vi "FPGAinit.vi"(4 "Testpulse Cluster":T3={"Master Pulser On/Off"=FALSE, "Testpulse Turnaround Time (samples)"=14, "Pulse Separation (samples)"=0, "Pulse duration (samples)"=0}, 5 "DAQ Info Cluster":T2={"Data Chunks per File"=1000, "Samples per Waveform"=95, "Pretrigger Samples"=15, "circular buffer length (samples)"=1000, "Waveforms per Data Chunk"=5000} {"Waveforms per Data Chunk" format="%.2p"}, 6 "Channel Cluster":T1={"det_type"=["", "", "", "", "", "", "", ""], "Serial numbers"=["", "", "", "", "", "", "", ""], "Sources"=["", "", "", "", "", "", "", ""], "Trigger level"=[4000, 4000, 4000, 4000, 4000, 4000, 4000, 4000], "Data Record On/Off"=[FALSE, FALSE, FALSE, FALSE, FALSE, FALSE, FALSE, FALSE], "Number of Channels"=8}, 7 "General Cluster":cluster{"Location":i16} {"Location" items=["Purdue", "NIKHEF", "Zurich", "???"]}, 8 "error in":errorcluster, 11 "FPGA VI Reference In":refnum<k20>) -> (0 "error out":errorcluster, 3 "FPGA VI Reference Out":refnum<k20>)   [LabVIEW 2012]
uses:
  <vilib>/FPGAPlugInAG/Dynamic/niLvFpga_Reset_Dynamic.vi
  <vilib>/Utility/error.llb/Error Cluster From Error Code.vi
  <vilib>/LabVIEW Targets/FPGA/FlexRIO/CustomFPGAMethods/79XXR_Method_IOModuleStatusImpl.vi
  <vilib>/FPGAPlugInAG/Dynamic/niLvFpga_Run_Dynamic.vi
  <vilib>/rvi/errors/niLvFpgaAdjustHostInterfaceError.vi
  <vilib>/rvi/interface/nirviMethod/nirviMethod.xnode
  <vilib>/rvi/interface/nirviReadWriteControl/nirviReadWriteControl.xnode
  <vilib>/rvi/errors/niLvFpgaMergeErrorWithErrorCode.vi
  <vilib>/rvi/interface/Simulation/niFpgaSimulationCallBeginRW.vi
  NiFpgaLv.dll
  <vilib>/FPGAPlugInAG/Dynamic/niLvFpga_ConfigureFifo_Dynamic.vi
  <vilib>/FPGAPlugInAG/Dynamic/niLvFpga_StartFifo_Dynamic.vi
panel:
  # "Channel 0"
  # "Channel 1"
  # "Channel 2"
  # "Channel 3"
  # "Channel 4"
  # "Channel 5"
  # "Channel 6"
  # "Channel 7"
  # "Waveform/Data Chunk information"
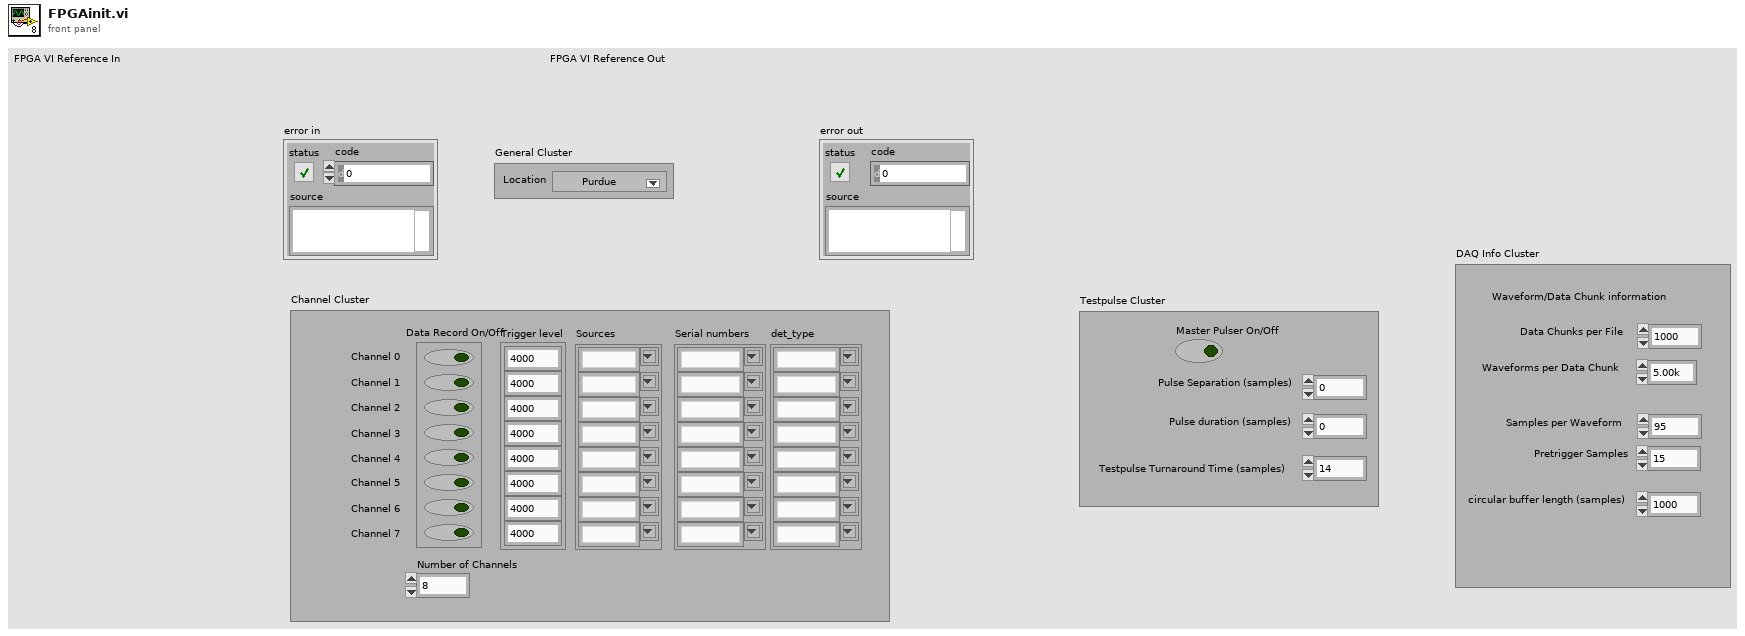
[diagram p1: front panel]
types:
  T1 = cluster{"det_type":string[], "Serial numbers":string[], "Sources":string[], "Trigger level":i16[], "Data Record On/Off":bool[], "Number of Channels":u8}
  T2 = cluster{"Data Chunks per File":u32, "Samples per Waveform":u32, "Pretrigger Samples":u32, "circular buffer length (samples)":u32, "Waveforms per Data Chunk":u32}
  T3 = cluster{"Master Pulser On/Off":bool, "Testpulse Turnaround Time (samples)":u32, "Pulse Separation (samples)":u32, "Pulse duration (samples)":u32}
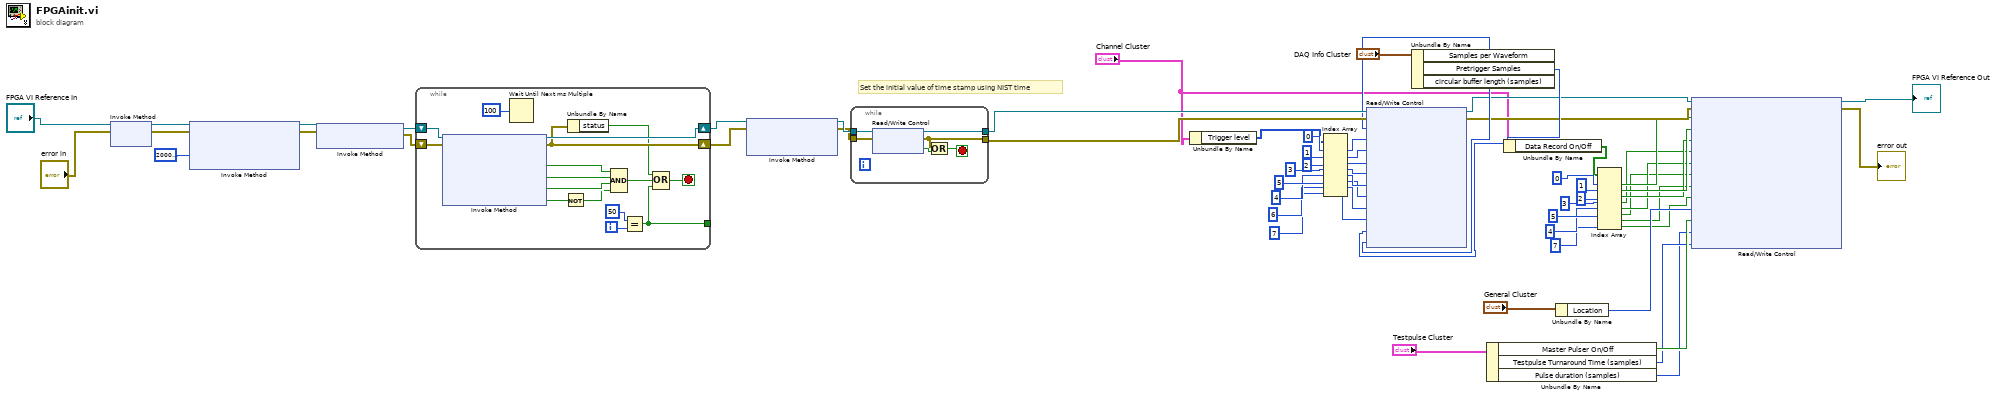
[diagram p0: block diagram]
diagram:
  # "Set the initial value of time stamp using NIST time"
  n1 = xnode "Invoke Method"("FPGA VI Reference In"="FPGA VI Reference In", "error in"="error in") -> ("FPGA VI Reference Out"=w48:refnum<k20>, "error out"=w47:errorcluster)
  n2 = xnode "Invoke Method"("FPGA VI Reference In"=w48, "error in"=w47, "Requested Depth"=u32 20000000) -> ("FPGA VI Reference Out"=w51:refnum<k20>, "error out"=w50:errorcluster)  [unwired: 1 out]
  n3 = xnode "Invoke Method"("FPGA VI Reference In"=w51, "error in"=w50) -> ("FPGA VI Reference Out"=w59:refnum<k20>, "error out"=w58:errorcluster)
  n4 = while {
    shift-right: [w70] -> w52
    shift-left: w58 -> [w78]
    shift-right: [w77] -> w53
    shift-left: w59 -> [w79]
    tunnel: [w66] -> _
    i -> [w72]
    stop <- w67 stop-if-true
    n5 = xnode "Invoke Method"("FPGA VI Reference In"=w79, "error in"=w78) -> ("FPGA VI Reference Out"=w77:refnum<k20>, "error out"=w70:errorcluster, "IO Module Present?"=w76:bool, "Power Enabled?"=w75:bool, "IO Enabled?"=w74:bool, "IO Module Mismatch?"=w65:bool)
    n6 = Wait Until Next ms Multiple(millisecond multiple=u32 100) -> ()  [unwired: 1 out]
    n7 = Not(x=w65) -> (.not. x?=w64:bool)
    n8 = Unbundle By Name(w70) -> ("status"=w69:bool)
    n9 = Compound Arithmetic op=AND(w76, w75, w74, w64) -> (w68:bool)
    n10 = Equal?(x=50, y=w72) -> (x = y?=w66:bool)
    n11 = Compound Arithmetic op=OR(w69, w68, w66) -> (w67:bool)
  }
  n12 = xnode "Invoke Method"("FPGA VI Reference In"=w53, "error in"=w52) -> ("FPGA VI Reference Out"=w62:refnum<k20>, "error out"=w61:errorcluster)  [unwired: 1 in]
  n13 = while {
    tunnel: [w80] -> w45
    tunnel: [w85] -> w46
    tunnel: w62 -> [w84]
    tunnel: w61 -> [w83]
    stop <- w81 stop-if-true
    n14 = xnode "Read/Write Control"("FPGA VI Reference In"=w84, "error in"=w83) -> ("FPGA VI Reference Out"=w85:refnum<k20>, "error out"=w80:errorcluster, "Init Done"=w82:bool)
    n15 = Or(x=w80, y=w82) -> (x .or. y?=w81:bool)
  }
  n16 = Unbundle By Name("Channel Cluster") -> ("Trigger level"=w57:i16[])
  n17 = Index Array(array=w57, index #1=0 ("index"), index #2=1 ("index"), index #3=2 ("index"), index #4=3 ("index"), index #5=4 ("index"), index #6=5 ("index"), index #7=6 ("index"), index #8=7 ("index")) -> (element #1=w44:i16, element #2=w23:i16, element #3=w22:i16, element #4=w21:i16, element #5=w20:i16, element #6=w19:i16, element #7=w18:i16, element #8=w17:i16)
  n18 = Unbundle By Name("DAQ Info Cluster") -> ("Samples per Waveform"=w41:u32, "Pretrigger Samples"=w42:u32, "circular buffer length (samples)"=w43:u32)
  n19 = xnode "Read/Write Control"("FPGA VI Reference In"=w46, "error in"=w45, "Record Size only data"=w41, "Trigger 0"=w44, "Trigger 1"=w23, "Trigger 2"=w22, "Trigger 3"=w21, "Trigger 4"=w20, "Trigger 5"=w19, "Trigger 6"=w18, "Trigger 7"=w17, "# of pretrigger"=w42, "circular buffer length"=w43) -> ("FPGA VI Reference Out"=w40:refnum<k20>, "error out"=w38:errorcluster)
  n20 = Unbundle By Name("Testpulse Cluster") -> ("Master Pulser On/Off"=w36:bool, "Testpulse Turnaround Time (samples)"=w35:u32, "Pulse duration (samples)"=w34:u32)
  n21 = Unbundle By Name("Channel Cluster") -> ("Data Record On/Off"=w9:bool[])
  n22 = Unbundle By Name("General Cluster") -> ("Location"=w37:i16)
  n23 = Index Array(array=w9, index #1=0 ("index"), index #2=1 ("index"), index #3=2 ("index"), index #4=3 ("index"), index #5=4 ("index"), index #6=5 ("index"), index #8=7 ("index")) -> (element #1=w8:bool, element #2=w7:bool, element #3=w6:bool, element #4=w5:bool, element #5=w4:bool, element #6=w3:bool, element #7=w2:bool, element #8=w1:bool)  [unwired: 1 in]
  n24 = xnode "Read/Write Control"("FPGA VI Reference In"=w40, "error in"=w38, "channel 0 on/off"=w8, "channel 1 on/off"=w7, "channel 2 on/off"=w6, "channel 3 on/off"=w5, "channel 4 on/off"=w4, "channel 5 on/off"=w3, "channel 6 on/off"=w2, "channel 7 on/off"=w1, "location"=w37, "Testpulser On/Off"=w36, "Testpulse duration (20 ns ticks)"=w34, "Testpulse Time Delay (20 ns ticks)"=w35) -> ("FPGA VI Reference Out"=→"FPGA VI Reference Out":refnum<k20>, "error out"=→"error out":errorcluster)
